vi "Get Section Scalars.vi"(8 "error in":errorcluster, 11 "section ref in":T1 format="%.0x") -> (0 "error out":errorcluster, 2 "section scalars out":T2[](array[typedef]), 3 "section ref in":T1 format="%.0x")   [LabVIEW 2018]
uses:
  Addon Shared/Types/Data Type.ctl
  Addon Shared/FPGA Addon Shared.lvlib
  APIs/Scripting API/TypeDefs/Output Scalar Data.ctl
  APIs/Scripting API/Scripting API.lvlib
  Addon Shared/Types/FG Action.ctl
  <vilib>/NI Veristand/Custom Device API/Custom Device API.lvlib
  Addon Shared/Types/Register Information.ctl
  <vilib>/NI Veristand/Custom Device API/Custom Device Item Ref.ctl
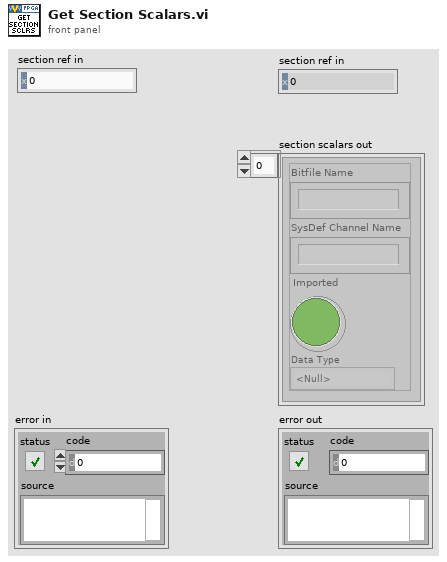
[diagram p1: front panel]
types:
  T1 = typedef "Custom Device API.lvlib/Custom Device Item Ref.ctl" = u64
  T2 = typedef "Scripting API.lvlib/Output Scalar Data.ctl" = cluster{"Bitfile Name":string, "SysDef Channel Name":string, "Imported":bool, "Data Type":T3}
  T3 = typedef "FPGA Addon Shared.lvlib/Data Type.ctl" = enum8{"<Null>", "I8", "I16", "I32", "I64", "U8", "U16", "U32", "U64", "SGL", "Boolean", "Analog PWM In Settings", "Analog PWM In", "Digital PWM In Settings", "Digital PWM In", "Digital PWM Out", "Sine Out", "FXP+/-24.5", "FXP+/-16.5", "FXP+/-32.8", "FXP+/-64.32", "FXP+/-16.7", "FXP+/-20.5", "FXP+/-27.5", "FXP+/-32.16", "FXP+16.3", "FXP+18.3", "Digital Static In", "Digital Static Out", "Digital Static In Settings", "Digital WSS Out", "Quad Encoder Settings", "Quad Encoder In", "Group"}
  T4 = typedef "FPGA Addon Shared.lvlib/FG Action.ctl" = enum8{"GET", "SET"}
  T5 = typedef "FPGA Addon Shared.lvlib/Register Information.ctl" = cluster{"Name":string, "Data Type":T3, "Default Value":variant}
  T6 = typedef "Custom Device API.lvlib/Custom Device Item Info.ctl" = cluster{"Name":string, "Is Channel":bool, "GUID":string, "Is Waveform":bool}
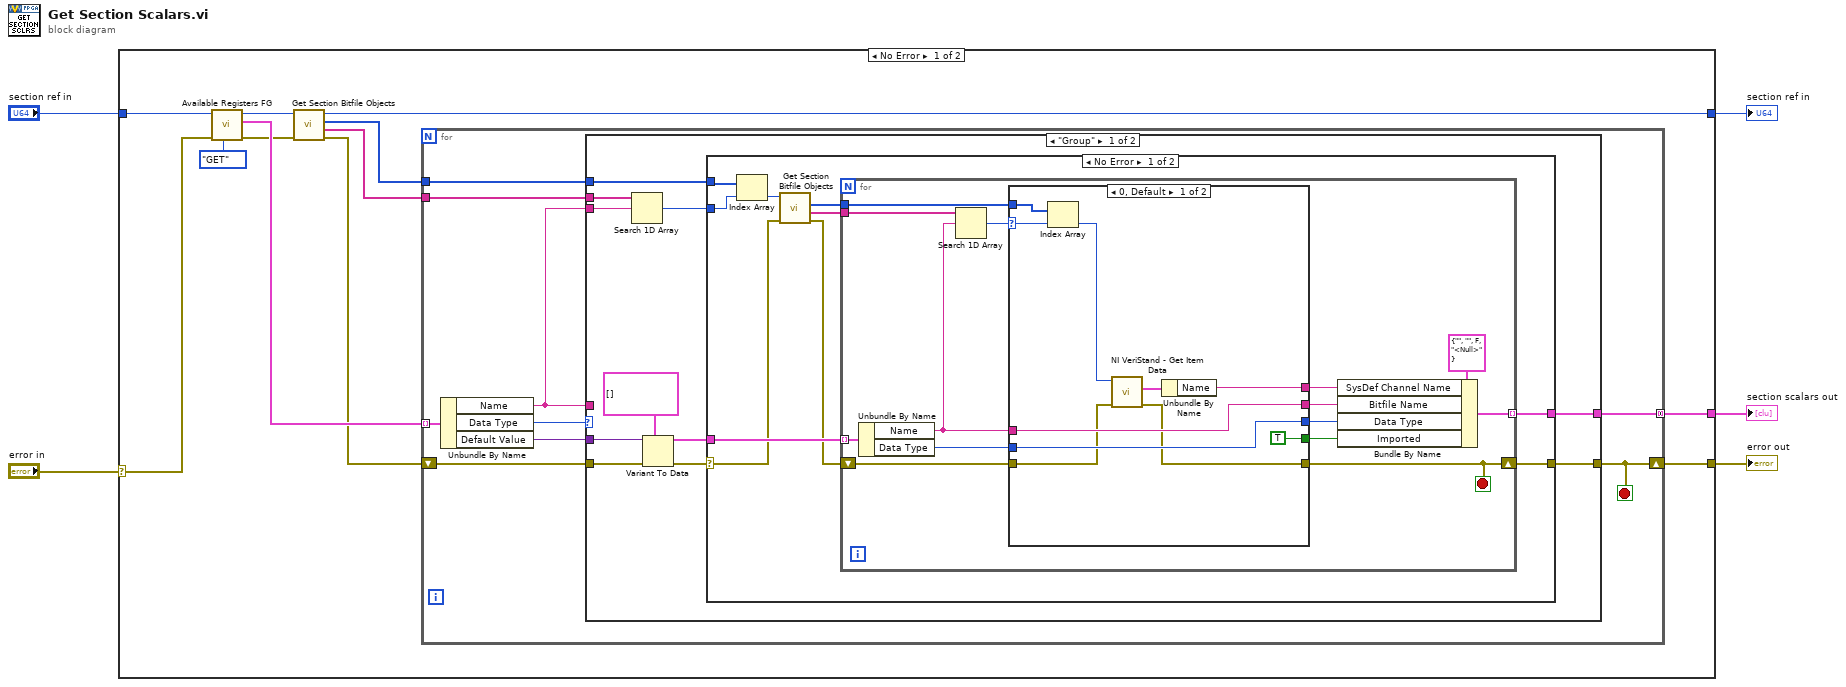
[diagram p0: block diagram]
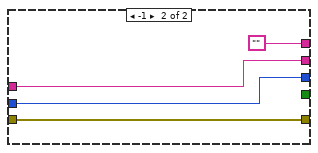
[diagram p2: hidden frame]
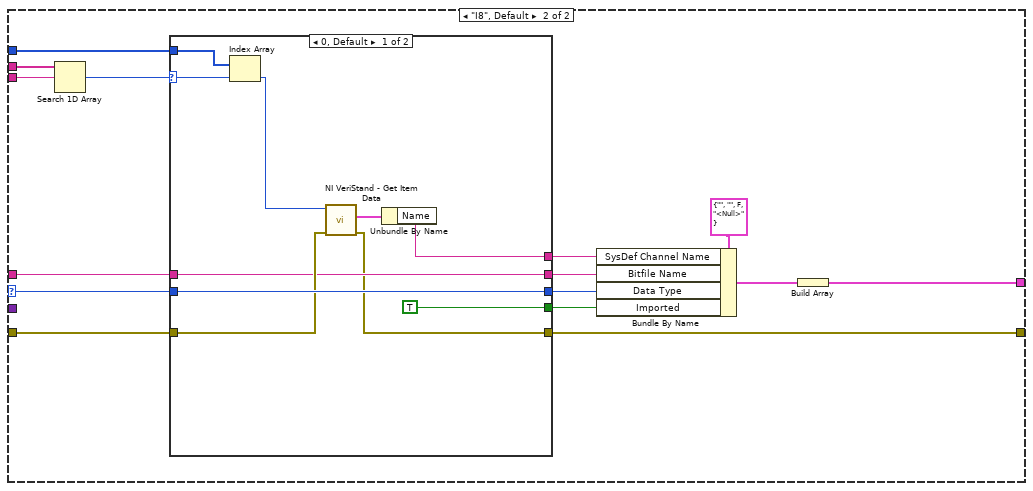
[diagram p4: hidden frame]
diagram:
  n1 = case shown="No Error" "error in" {
    selector: "error in" -> [w8 w106]
    tunnel: "section ref in" -> [w15 w105]
    tunnel: [w7 w105] -> w4
    tunnel: [w10 w106] -> w2
    tunnel: [w9 _] -> w1
    frame No Error {
      n2 = call "Available Registers FG.vi"("Action"=FG_Action."GET", "error in (no error)"=w8, "Item Ref"=w15) -> ("error out"=w12:errorcluster, "Available Registers"=w17:T5[], "Item Ref out"=w16:T1)  [unwired: 6 in]
      n3 = call "Get Section Bitfile Objects.vi"("error in"=w12, "item ref in"=w16) -> ("error out"=w11:errorcluster, "bitfile object names"=w13:string[], "section children refs"=w6:T1[], "item ref out"=w7:T1)  [unwired: 6 in]
      n4 = for {
        tunnel: w13 -> [w23]
        tunnel: w17 -> [w26] mode=indexing
        shift-right: [w18] -> w10
        shift-left: w11 -> [w21]
        tunnel: w6 -> [w24]
        tunnel: [w19] -> w9 mode=concatenating
        stop <- w18 stop-if-true
        n5 = Unbundle By Name(w26) -> ("Name"=w22:string, "Data Type"=w25:T3, "Default Value"=w20:variant)
        n6 = case shown="\"Group\"" w25 {
          selector: w25 -> [_ w83]
          tunnel: w24 -> [w30 w88]
          tunnel: w22 -> [w31 w91]
          tunnel: w23 -> [w32 w90]
          tunnel: w22 -> [_ w87]
          tunnel: w21 -> [w37 w82]
          tunnel: [w28 w79] -> w18
          tunnel: w20 -> [w36 _]
          tunnel: [w27 w77] -> w19
          frame "Group" {
            n7 = Search 1D Array(1D array=w32, element=w31) -> (index of element=w29:i32)  [unwired: 1 in]
            n8 = Variant To Data(error in=w37, type=T5[] [], Variant=w36) -> (data=w34:T5[], error out=w33:errorcluster)
            n9 = case shown="No Error" w33 {
              selector: w33 -> [w39 w76]
              tunnel: w34 -> [w47 _]
              tunnel: w30 -> [w46 _]
              tunnel: w29 -> [w45 _]
              tunnel: [w41 w76] -> w28
              tunnel: [w40 _] -> w27
              frame No Error {
                n10 = Index Array(array=w46, index=w45) -> (element=w44:T1)
                n11 = call "Get Section Bitfile Objects.vi"("error in"=w39, "item ref in"=w44) -> ("error out"=w38:errorcluster, "bitfile object names"=w43:string[], "section children refs"=w42:T1[])  [unwired: 6 in, 1 out]
                n12 = for {
                  tunnel: w47 -> [w61] mode=indexing
                  tunnel: w43 -> [w60]
                  tunnel: w42 -> [w49]
                  shift-right: [w50] -> w41
                  shift-left: w38 -> [w53]
                  tunnel: [w51] -> w40 mode=indexing
                  stop <- w50 stop-if-true
                  n13 = Unbundle By Name(w61) -> ("Name"=w57:string, "Data Type"=w59:T3)
                  n14 = Search 1D Array(1D array=w60, element=w57) -> (index of element=w48:i32)  [unwired: 1 in]
                  n15 = case shown="0, Default" w48 {
                    selector: w48 -> [w62 _]
                    tunnel: w59 -> [w69 w74]
                    tunnel: w57 -> [w70 w75]
                    tunnel: [w70 w75] -> w56
                    tunnel: [w69 w74] -> w55
                    tunnel: [TRUE ("Imported?") _] -> w54
                    tunnel: w53 -> [w67 w73]
                    tunnel: [w66 ""] -> w52
                    tunnel: [w65 w73] -> w50
                    tunnel: w49 -> [w64 _]
                    frame 0, Default {
                      n16 = Index Array(array=w64, index=w62) -> (element=w63:T1)
                      n17 = call <vilib>:"NI VeriStand - Get Item Data.vi"("error in (no error)"=w67, "Item Ref in"=w63) -> ("error out"=w65:errorcluster, "Item Info"=w71:T6)  [unwired: 6 in, 2 out]
                      n18 = Unbundle By Name(w71) -> ("Name"=w66:string)
                    }
                    frame -1 {
                    }
                  }
                  n19 = Bundle By Name(cluster=T2 {"Bitfile Name"="", "SysDef Channel Name"="", "Imported"=FALSE, "Data Type"=enum."<Null>"} ("Scalar data"), "SysDef Channel Name"=w52, "Bitfile Name"=w56, "Data Type"=w55, "Imported"=w54) -> (w51:T2)
                }
              }
              frame Error {
              }
            }
          }
          frame "I8", Default {
            n20 = Search 1D Array(1D array=w90, element=w91) -> (index of element=w89:i32)  [unwired: 1 in]
            n21 = case shown="0, Default" w89 {
              selector: w89 -> [w100 _]
              tunnel: w88 -> [w101 _]
              tunnel: w87 -> [w93 w104]
              tunnel: [w97 _] -> w85
              tunnel: [w96 w103] -> w84
              tunnel: w83 -> [w96 w103]
              tunnel: w82 -> [w95 w102]
              tunnel: [TRUE _] -> w81
              tunnel: [w93 w104] -> w80
              tunnel: [w92 w102] -> w79
              frame 0, Default {
                n22 = Index Array(array=w101, index=w100) -> (element=w99:T1)
                n23 = call <vilib>:"NI VeriStand - Get Item Data.vi"("error in (no error)"=w95, "Item Ref in"=w99) -> ("error out"=w92:errorcluster, "Item Info"=w98:T6)  [unwired: 6 in, 2 out]
                n24 = Unbundle By Name(w98) -> ("Name"=w97:string)
              }
              frame -1 {
              }
            }
            n25 = Bundle By Name(cluster=T2 {"Bitfile Name"="", "SysDef Channel Name"="", "Imported"=FALSE, "Data Type"=enum."<Null>"} ("Scalar data"), "SysDef Channel Name"=w85, "Bitfile Name"=w80, "Data Type"=w84, "Imported"=w81) -> (w78:T2)
            n26 = Build Array(w78) -> (w77:T2[])
          }
        }
      }
    }
    frame Error {
    }
  }
  "section scalars out" <- w1
  "section ref in" <- w4
  "error out" <- w2
